vi "DAQ Sin wave read write.vi"() -> ()   [LabVIEW 2020]
uses:
  <vilib>/DAQmx/read.llb/DAQmx Read (Analog DBL 1Chan 1Samp).vi
  <vilib>/DAQmx/write.llb/DAQmx Write (Analog DBL 1Chan 1Samp).vi
  <vilib>/DAQmx/create/channels.llb/DAQmx Create Channel (AO-Voltage-Basic).vi
  <vilib>/DAQmx/create/channels.llb/DAQmx Create Channel (AI-Voltage-Basic).vi
  <vilib>/DAQmx/miscellaneous.llb/DAQmx Fill In Error Info.vi
panel:
  in  "DAQmx Physical Channel 2":tag
  out "Slide":dbl(slide) scale=0.0..10.0
  out "Meter":dbl(knob) scale=0.0..8.0
  in  "stop":bool
  in  "DAQmx Physical Channel":tag
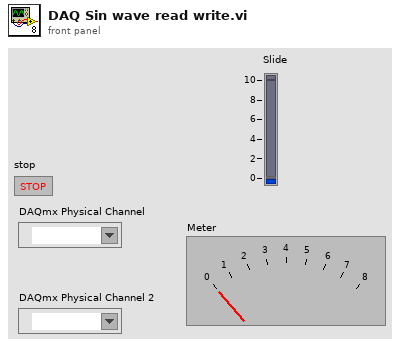
[diagram p1: front panel]
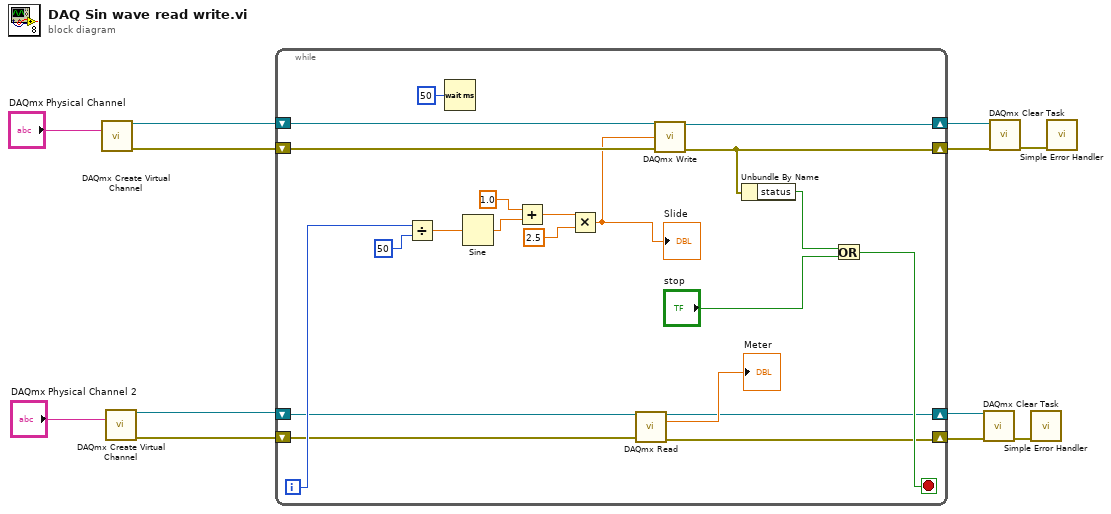
[diagram p0: block diagram]
diagram:
  n1 = call-poly <vilib>:"DAQmx Create Virtual Channel.vi"("physical channels"="DAQmx Physical Channel") -> ("task out"=w10:refnum<k21>, "error out"=w8:errorcluster)  [unwired: 13 in]
  n2 = call-poly <vilib>:"DAQmx Create Virtual Channel.vi"("physical channels"="DAQmx Physical Channel 2") -> ("task out"=w5:refnum<k21>, "error out"=w4:errorcluster)  [unwired: 13 in]
  n3 = while {
    shift-right: [w25] -> w9
    shift-left: w10 -> [w26]
    shift-right: [w21] -> w7
    shift-left: w8 -> [w24]
    shift-right: [w14] -> w3
    shift-left: w5 -> [w17]
    shift-right: [w13] -> w2
    shift-left: w4 -> [w16]
    i -> [w23]
    stop <- w18 stop-if-true
    n4 = Divide(x=w23, y=50) -> (x/y=w32:dbl)
    n5 = Wait (ms)(milliseconds to wait=u32 50) -> ()  [unwired: 1 out]
    n6 = Sine(x=w32) -> (sin(x)=w31:dbl)
    n7 = Add(x=1.0, y=w31) -> (x+y=w29:dbl)
    n8 = Multiply(x=w29, y=2.5) -> (x*y=w22:dbl)
    "Slide" <- w22
    n9 = call-poly <vilib>:"DAQmx Read.vi"("task/channels in"=w17, "error in"=w16) -> ("task out"=w14:refnum<k21>, "data"=→"Meter":dbl, "error out"=w13:errorcluster)  [unwired: 11 in]
    n10 = call-poly <vilib>:"DAQmx Write.vi"("task/channels in"=w26, "data"=w22, "error in"=w24) -> ("task out"=w25:refnum<k21>, "error out"=w21:errorcluster)  [unwired: 10 in, 1 out]
    n11 = Unbundle By Name(w21) -> ("status"=w20:bool)
    n12 = Or(x=w20, y="stop") -> (x .or. y?=w18:bool)
  }
  n13 = call <vilib>:"DAQmx Clear Task.vi"("task in"=w3, "error in"=w2) -> ("error out"=w1:errorcluster)  [unwired: 13 in]
  n14 = call <vilib>:"DAQmx Clear Task.vi"("task in"=w9, "error in"=w7) -> ("error out"=w11:errorcluster)  [unwired: 13 in]
  n15 = call <vilib>:"Simple Error Handler.vi"("error in (no error)"=w1) -> ()  [unwired: 4 in, 5 out]
  n16 = call <vilib>:"Simple Error Handler.vi"("error in (no error)"=w11) -> ()  [unwired: 4 in, 5 out]
